vi "Is FOOD in Snake.vi"(9 "Map width":i32, 10 "Map Length":i32, 11 "Snake Position":i32[][](array[numeric])) -> (2 "Boolean":bool, 3 "Food Position":i32[](array[numeric]))   [LabVIEW 2014]
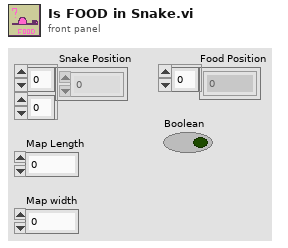
[diagram p1: front panel]
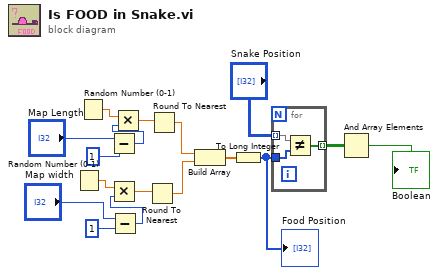
[diagram p0: block diagram]
diagram:
  n1 = Random Number (0-1)() -> (number: 0 to 1=w3:dbl)
  n2 = Random Number (0-1)() -> (number: 0 to 1=w1:dbl)
  n3 = Subtract(x="Map Length", y=i16 1) -> (x-y=w15:i32)
  n4 = Subtract(x="Map width", y=i16 1) -> (x-y=w13:i32)
  n5 = Multiply(x=w3, y=w13) -> (x*y=w4:dbl)
  n6 = Multiply(x=w1, y=w15) -> (x*y=w2:dbl)
  n7 = Round To Nearest(number=w4) -> (nearest integer value=w6:dbl)
  n8 = Round To Nearest(number=w2) -> (nearest integer value=w5:dbl)
  n9 = Build Array(w5, w6) -> (w7:dbl[])
  n10 = To Long Integer(number=w7) -> (32bit integer=w11:i32[])
  "Food Position" <- w11
  n11 = for {
    tunnel: w11 -> [w19]
    tunnel: "Snake Position" -> [w20] mode=indexing
    tunnel: [w18] -> w9 mode=indexing
    n12 = Not Equal?(x=w20, y=w19) -> (x != y?=w18:bool[])
  }
  n13 = And Array Elements(Boolean array=w9) -> (logical AND=→"Boolean":bool)
